vi "FTW-JSON-Escape.vi"(1 "String":string) -> (0 "Escaped UTF-8 String":string)   [LabVIEW 2014]
panel:
  # "Inputs"
  # "Outputs"
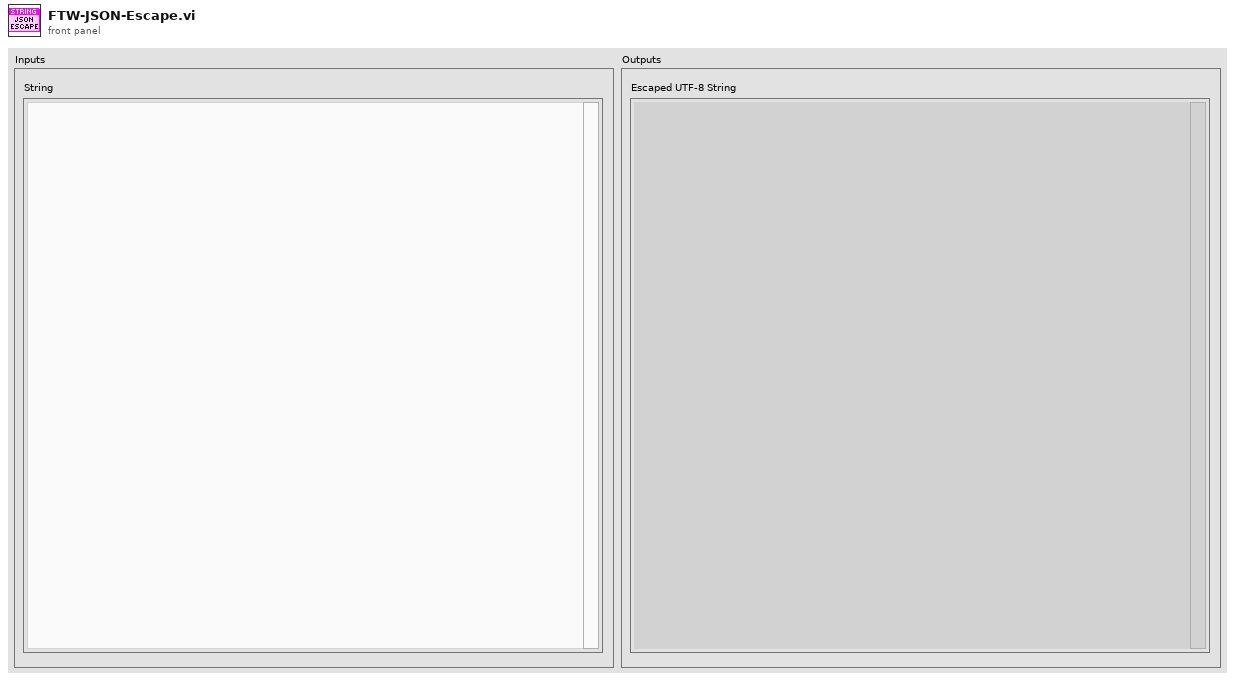
[diagram p1: front panel]
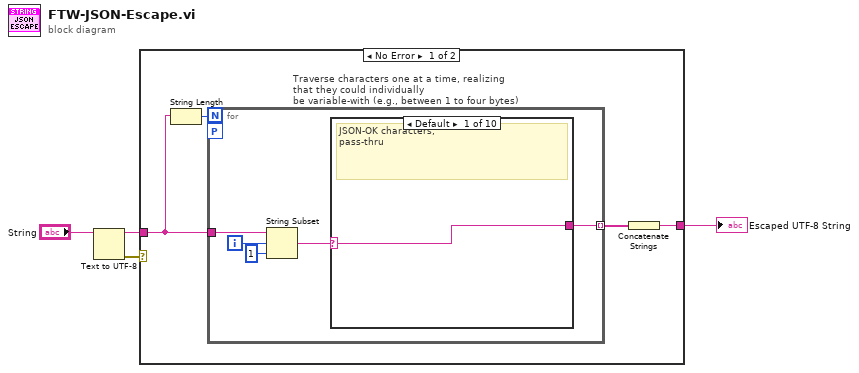
[diagram p0: block diagram]
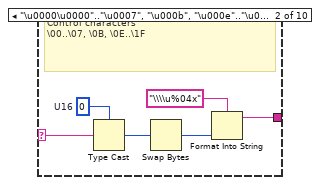
[diagram p2: hidden frame]
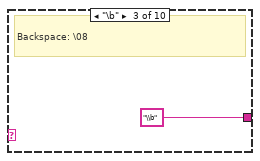
[diagram p3: hidden frame]
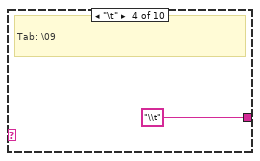
[diagram p4: hidden frame]
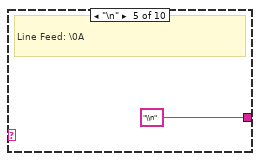
[diagram p5: hidden frame]
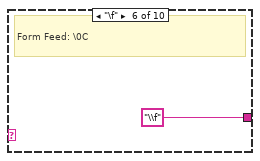
[diagram p6: hidden frame]
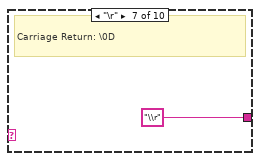
[diagram p7: hidden frame]
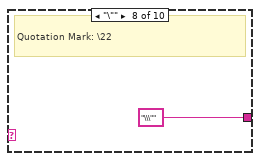
[diagram p8: hidden frame]
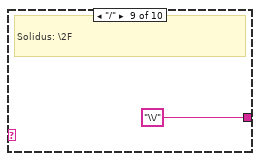
[diagram p9: hidden frame]
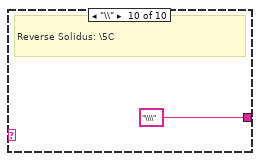
[diagram p10: hidden frame]
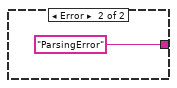
[diagram p11: hidden frame]
diagram:
  n1 = Text to UTF-8(11:"String") -> (0:w1:errorcluster, 3:w2:string)  [unwired: 2 in]
  n2 = case shown="No Error" w1 {
    tunnel: [w7 "ParsingError" ("Escaped String")] -> w4
    tunnel: w2 -> [w6 _]
    frame No Error {
      n3 = String Length(string=w6) -> (length=w5:i32)
      n4 = for "Traverse characters one at a time, realizing that they could individually\nbe variable-with (e.g., between 1 to four bytes)" {
        N: w5 -> [_]
        tunnel: [w13] -> w8 mode=indexing
        tunnel: w6 -> [w12]
        workers-P: _ -> [_]
        i -> [w11]
        n5 = String Subset(string=w12, offset (0)=w11, length (rest)=1 ("length (rest)")) -> (substring=w9:string)
        n6 = case shown="Default" w9 {
          selector: w9 -> [w14 w18 _ _ _ _ _ _ _ _]
          tunnel: [w14 w19 "\\b" "\\t" "\\n" "\\f" "\\r" "\\\"" "\\/" "\\\\"] -> w13
          frame Default {
            # "JSON-OK characters;\npass-thru"
          }
          frame "\u0000\u0000".."\u0007", "\u000b", "\u000e".."\u001f" {
            w17 = u16 0  # U16
            # "Control characters\n\\00..\\07, \\0B, \\0E..\\1F"
            n7 = Type Cast(type=w17, x=w18) -> (*(type *) &x=w16:u16)
            n8 = Swap Bytes(anything=w16) -> (byte swapped=w15:u16)
            n9 = Format Into String(format string="\\\\u%04x", w15) -> (resulting string=w19:string)  [unwired: 2 in, 1 out]
          }
          frame "\b" {
            # "Backspace: \\08"
          }
          frame "\t" {
            # "Tab: \\09"
          }
          frame "\n" {
            # "Line Feed: \\0A"
          }
          frame "\f" {
            # "Form Feed: \\0C"
          }
          frame "\r" {
            # "Carriage Return: \\0D"
          }
          frame "\"" {
            # "Quotation Mark: \\22"
          }
          frame "/" {
            # "Solidus: \\2F"
          }
          frame "\\" {
            # "Reverse Solidus: \\5C"
          }
        }
      }
      n10 = Concatenate Strings(w8) -> (w7:string)
    }
    frame Error {
    }
  }
  "Escaped UTF-8 String" <- w4
